vi "Get NIPM CLI Full Path.vi"(8 "error in (no error)":errorcluster) -> (0 "error out":errorcluster, 3 "NIPM CLI":path)   [LabVIEW 2021, in "NIPM_API.lvlib"]
doc: "Returns the full path of nipkg.exe for the current installation of NI Package Manager on the system."
uses:
  NIPM_API.lvlib
  <vilib>/registry/registry.llb/Registry SAM.ctl
  <vilib>/registry/registry.llb/Registry RtKey.ctl
  <vilib>/registry/registry.llb/Read Registry Value Simple STR.vi
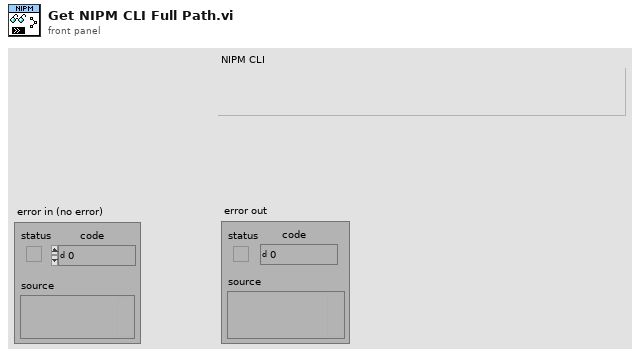
[diagram p1: front panel]
types:
  T1 = typedef "Registry RtKey.ctl" = enum32{"HKEY_CLASSES_ROOT", "HKEY_CURRENT_USER", "HKEY_LOCAL_MACHINE", "HKEY_USERS", "HKEY_PERFORMANCE_DATA", "HKEY_CURRENT_CONFIG", "HKEY_DYN_DATA"}
  T2 = typedef "Registry SAM.ctl" = enum32{"KEY_QUERY_VALUE", "KEY_SET_VALUE", "KEY_CREATE_SUB_KEY", "KEY_ENUMERATE_SUB_KEYS", "KEY_NOTIFY", "KEY_CREATE_LINK", "KEY_READ", "KEY_WRITE", "KEY_ALL_ACCESS", "KEY_READ | KEY_WRITE"}
  T3 = typedef "Registry refnum.ctl" = refnum<k1>
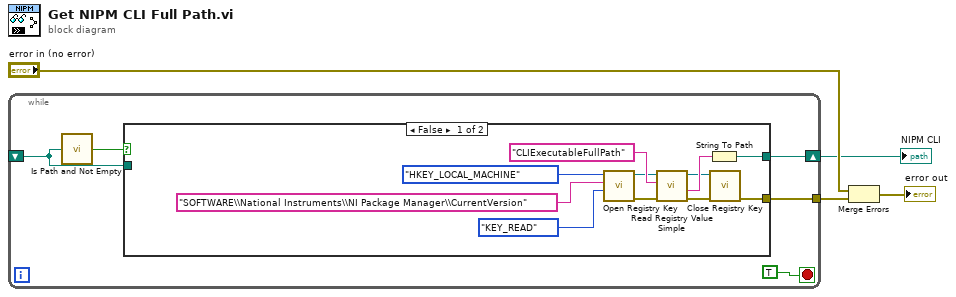
[diagram p0: block diagram]
diagram:
  n1 = while {
    tunnel: [w9] -> w1
    shift-right: [w8] -> w2
    shift-left: _ -> [w5]
    stop <- TRUE stop-if-true
    n2 = call <vilib>:"Is Path and Not Empty.vi"("path"=w5) -> ("Is Path and Not Empty?"=w6:bool)  [unwired: 4 in]
    n3 = case shown="False" w6 {
      tunnel: [w20 _] -> w9
      tunnel: [w19 w21] -> w8
      tunnel: w5 -> [_ w21]
      frame False {
        n4 = call <vilib>:"Open Registry Key.vi"("security access mask (KEY_READ | KEY_WRITE)"=Registry_SAM."KEY_READ", "subkey"="SOFTWARE\\National Instruments\\NI Package Manager\\CurrentVersion", "root key (HKEY_LOCAL_MACHINE)"=Registry_RtKey."HKEY_LOCAL_MACHINE") -> ("error out"=w14:errorcluster, "refnum out"=w13:T3)  [unwired: 7 in]
        n5 = call-poly <vilib>:"Read Registry Value Simple.vi"("error in (no error)"=w14, "value"="CLIExecutableFullPath", "refnum"=w13) -> ("error out"=w17:errorcluster, "String/Binary data"=w18:string, "refnum out"=w16:T3)  [unwired: 3 in, 1 out]
        n6 = String To Path(string=w18) -> (path=w19:path)
        n7 = call <vilib>:"Close Registry Key.vi"("error in (no error)"=w17, "refnum"=w16) -> ("error out"=w20:errorcluster)  [unwired: 5 in]
      }
      frame True {
      }
    }
  }
  "NIPM CLI" <- w2
  n8 = Merge Errors("error in (no error)", w1) -> (→"error out":errorcluster)
